vi "PhaseCalibration.vi"(0 "Global Parameters":T1={"DC AI Min (V)"=0.0015, "DC AI Max (V)"=0.06, "Mixer AI Min (V)"=-0.3, "Mixer AI Max (V)"=0.3, "Bias AO Min (V)"=-1.0, "Bias AO Max (V)"=7.0, "Scan AO Min (V)"=-10.0, "Scan AO Max (V)"=10.0, "Fast Samp Freq (Hz)"=2500000.0, "Slow Samp Freq (Hz)"=250000.0}, 1 "Bias Voltages":dbl[](array[numeric]), 2 "LaserRepRate":dbl=80000000.0, 5 "Calibration Parameters":T2={"Target Lifetime (s)"=4e-09, "Integration Time (s)"=0.1, "Calibration Steps"=500.0}, 7 "Mixer1 Values":dbl[](array[numeric]), 9 "Mixer2 Values":dbl[](array[numeric]), 11 "Mixer3 Values":dbl[](array[numeric]), 12 "Mixer4 Values":dbl[](array[numeric]), 13 "[V_DC]":dbl, 14 "[O_B]":dbl) -> (4 "Mixer Phases":cluster{"Bias voltage":dbl[], dbl[]}[](array[cluster]), 6 "Calibrated Bias Voltages":dbl[](array[numeric]) caption="Calibrated bias voltage", 8 "[M/B]":dbl, 10 "[V_IF_max]":dbl, 15 "[V_IF_min]":dbl)   [LabVIEW 2018]
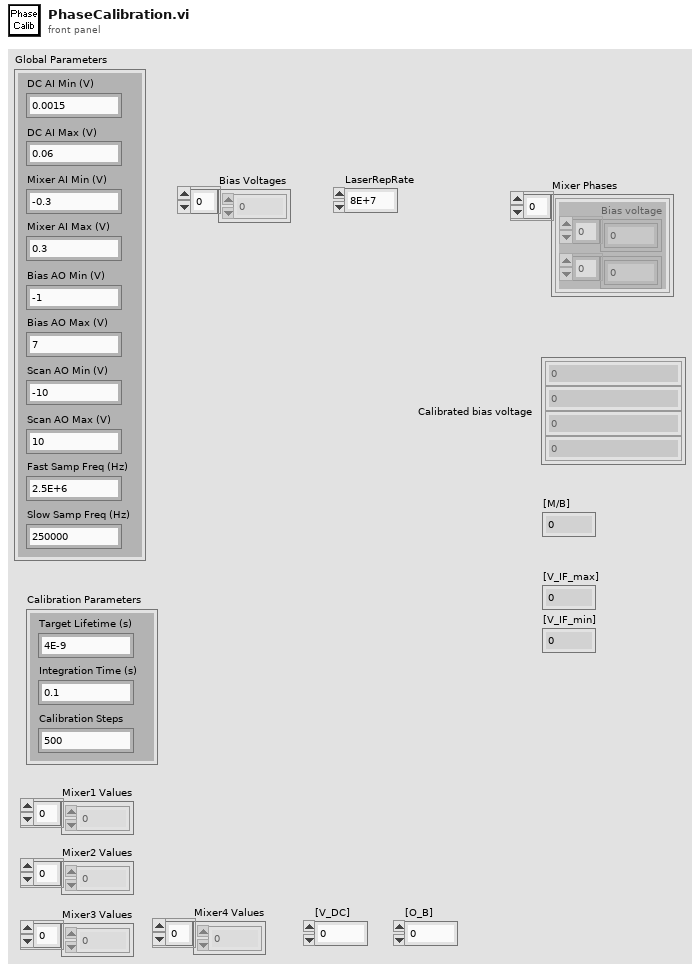
[diagram p1: front panel]
types:
  T1 = cluster{"DC AI Min (V)":dbl, "DC AI Max (V)":dbl, "Mixer AI Min (V)":dbl, "Mixer AI Max (V)":dbl, "Bias AO Min (V)":dbl, "Bias AO Max (V)":dbl, "Scan AO Min (V)":dbl, "Scan AO Max (V)":dbl, "Fast Samp Freq (Hz)":dbl, "Slow Samp Freq (Hz)":dbl}
  T2 = cluster{"Target Lifetime (s)":dbl, "Integration Time (s)":dbl, "Calibration Steps":dbl}
  T3 = cluster{"Bias Voltages":dbl[], "Phase Calibration Curve":dbl[]}
  T4 = cluster{"Bias Voltages":dbl[], "Phase Calibration Curve":dbl[]}[]
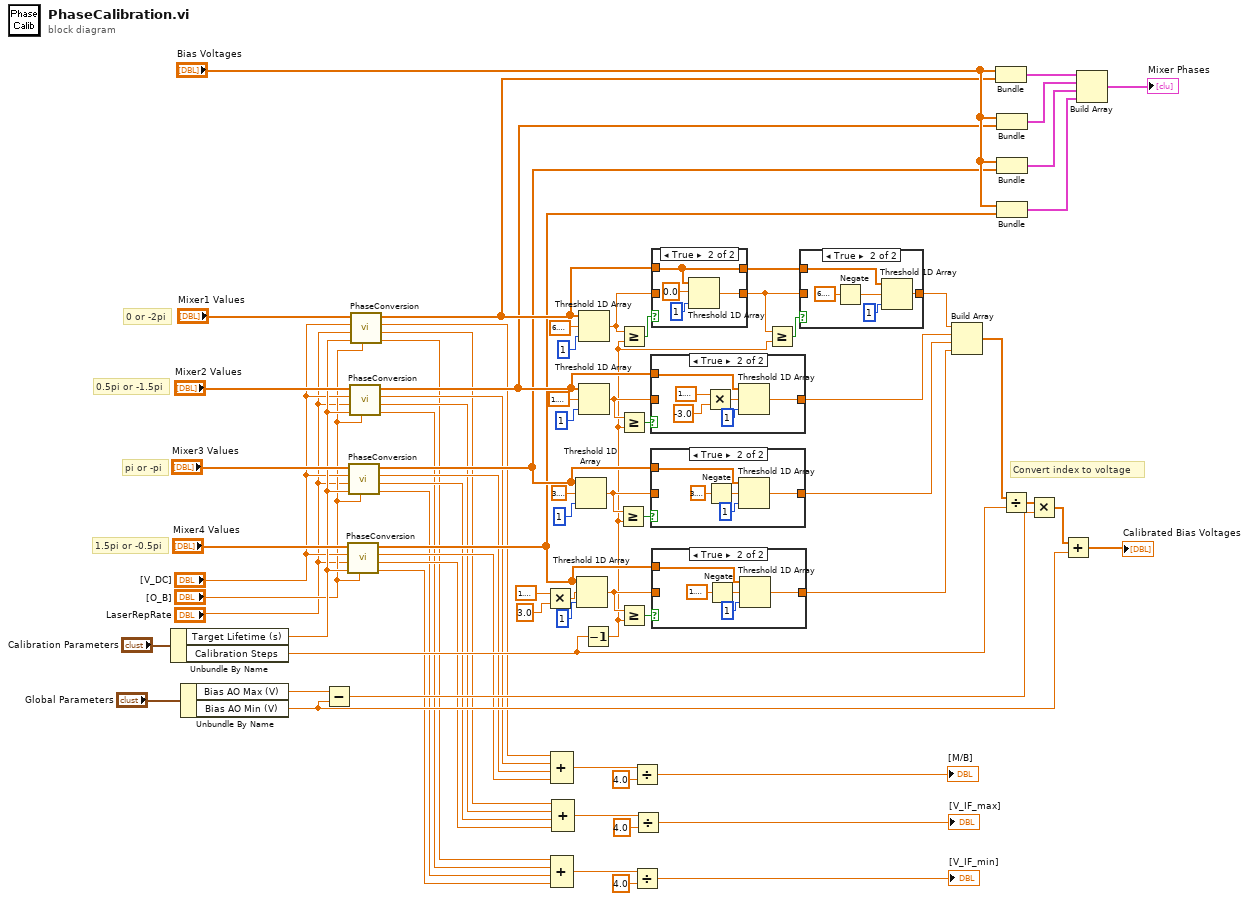
[diagram p0: block diagram]
diagram:
  # "Convert index to voltage"
  # "1.5pi or -0.5pi"
  # "pi or -pi"
  # "0.5pi or -1.5pi"
  # "0 or -2pi"
  n1 = Unbundle By Name("Calibration Parameters") -> ("Target Lifetime (s)"=w40:dbl, "Calibration Steps"=w61:dbl)
  n2 = Unbundle By Name("Global Parameters") -> ("Bias AO Max (V)"=w67:dbl, "Bias AO Min (V)"=w68:dbl)
  n3 = Subtract(x=w67, y=w68) -> (x-y=w72:dbl)
  n4 = call "PhaseConversion.vi"("[O_B]"="[O_B]", "Target Lifetime (s)"=w40, "Mod freq (Hz)"="LaserRepRate", "[V_DC]"="[V_DC]", "Mixer Values"="Mixer4 Values") -> ("V_IF_min"=w6:dbl, "V_IF_max"=w10:dbl, "M/B"=w27:dbl, "Phase Calibration Curve"=w41:dbl[])  [unwired: 2 in]
  n5 = call "PhaseConversion.vi"("[O_B]"="[O_B]", "Target Lifetime (s)"=w40, "Mod freq (Hz)"="LaserRepRate", "[V_DC]"="[V_DC]", "Mixer Values"="Mixer3 Values") -> ("V_IF_min"=w7:dbl, "V_IF_max"=w11:dbl, "M/B"=w26:dbl, "Phase Calibration Curve"=w42:dbl[])  [unwired: 2 in]
  n6 = call "PhaseConversion.vi"("[O_B]"="[O_B]", "Target Lifetime (s)"=w40, "Mod freq (Hz)"="LaserRepRate", "[V_DC]"="[V_DC]", "Mixer Values"="Mixer2 Values") -> ("V_IF_min"=w8:dbl, "V_IF_max"=w12:dbl, "M/B"=w25:dbl, "Phase Calibration Curve"=w43:dbl[])  [unwired: 2 in]
  n7 = call "PhaseConversion.vi"("[O_B]"="[O_B]", "Target Lifetime (s)"=w40, "Mod freq (Hz)"="LaserRepRate", "[V_DC]"="[V_DC]", "Mixer Values"="Mixer1 Values") -> ("V_IF_min"=w9:dbl, "V_IF_max"=w13:dbl, "M/B"=w24:dbl, "Phase Calibration Curve"=w44:dbl[])  [unwired: 2 in]
  n8 = Multiply(x=1.5707963267948966, y=3.0) -> (x*y=w57:dbl)
  n9 = Compound Arithmetic op=ADD(w24, w25, w26, w27) -> (w23:dbl)
  n10 = Compound Arithmetic op=ADD(w9, w8, w7, w6) -> (w15:dbl)
  n11 = Compound Arithmetic op=ADD(w13, w12, w11, w10) -> (w16:dbl)
  n12 = Threshold 1D Array(1:1 ("start index (0)"), 2:3.141592653589793, 3:w42) -> (0:w59:dbl)
  n13 = Threshold 1D Array(1:1 ("start index (0)"), 2:w57, 3:w41) -> (0:w53:dbl)
  n14 = Threshold 1D Array(1:1 ("start index (0)"), 2:6.283185307179586, 3:w44) -> (0:w49:dbl)
  n15 = Threshold 1D Array(1:1 ("start index (0)"), 2:1.5707963267948966, 3:w43) -> (0:w46:dbl)
  n16 = Decrement(x=w61) -> (x-1=w35:dbl)
  n17 = Greater Or Equal?(x=w59, y=w35) -> (x >= y?=w60:bool)
  n18 = Greater Or Equal?(x=w49, y=w35) -> (x >= y?=w50:bool)
  n19 = Greater Or Equal?(x=w46, y=w35) -> (x >= y?=w51:bool)
  n20 = Greater Or Equal?(x=w53, y=w35) -> (x >= y?=w54:bool)
  n21 = Divide(x=w23, y=4.0) -> (x/y=→"[M/B]":dbl)
  n22 = Divide(x=w15, y=4.0) -> (x/y=→"[V_IF_min]":dbl)
  n23 = Divide(x=w16, y=4.0) -> (x/y=→"[V_IF_max]":dbl)
  n24 = case shown="True" w51 {
    tunnel: [w76 w82] -> w45
    tunnel: w43 -> [_ w81]
    tunnel: w46 -> [w76 _]
    frame False {
    }
    frame True {
      n25 = Multiply(x=1.5707963267948966, y=-3.0) -> (x*y=w78:dbl)
      n26 = Threshold 1D Array(1:1 ("start index (0)"), 2:w78, 3:w81) -> (0:w82:dbl)
    }
  }
  n27 = case shown="True" w60 {
    tunnel: [w83 w88] -> w58
    tunnel: w59 -> [w83 _]
    tunnel: w42 -> [_ w85]
    frame False {
    }
    frame True {
      n28 = Negate(x=3.141592653589793) -> (-x=w87:dbl)
      n29 = Threshold 1D Array(1:1 ("start index (0)"), 2:w87, 3:w85) -> (0:w88:dbl)
    }
  }
  n30 = case shown="True" w50 {
    tunnel: [w90 w94] -> w34
    tunnel: w49 -> [w90 _]
    tunnel: w44 -> [w89 w92]
    tunnel: [w89 w92] -> w31
    frame False {
    }
    frame True {
      n31 = Threshold 1D Array(1:1 ("start index (0)"), 2:0.0 ("threshold y"), 3:w92) -> (0:w94:dbl)
    }
  }
  n32 = case shown="True" w54 {
    tunnel: [w95 w100] -> w52
    tunnel: w53 -> [w95 _]
    tunnel: w41 -> [_ w97]
    frame False {
    }
    frame True {
      n33 = Negate(x=1.5707963267948966) -> (-x=w99:dbl)
      n34 = Threshold 1D Array(1:1 ("start index (0)"), 2:w99, 3:w97) -> (0:w100:dbl)
    }
  }
  n35 = Greater Or Equal?(x=w34, y=w35) -> (x >= y?=w33:bool)
  n36 = case shown="True" w33 {
    tunnel: [w101 w106] -> w32
    tunnel: w34 -> [w101 _]
    tunnel: w31 -> [_ w104]
    frame False {
    }
    frame True {
      n37 = Negate(x=6.283185307179586) -> (-x=w102:dbl)
      n38 = Threshold 1D Array(1:1 ("start index (0)"), 2:w102, 3:w104) -> (0:w106:dbl)
    }
  }
  n39 = Build Array(w32, w45, w58, w52) -> (w29:dbl[])
  n40 = Bundle("Bias Voltages"="Bias Voltages", "Phase Calibration Curve"=w44) -> (w75:T3)  [unwired: 1 in]
  n41 = Bundle("Bias Voltages"="Bias Voltages", "Phase Calibration Curve"=w43) -> (w20:T3)  [unwired: 1 in]
  n42 = Bundle("Bias Voltages"="Bias Voltages", "Phase Calibration Curve"=w42) -> (w19:T3)  [unwired: 1 in]
  n43 = Bundle("Bias Voltages"="Bias Voltages", "Phase Calibration Curve"=w41) -> (w18:T3)  [unwired: 1 in]
  n44 = Divide(x=w29, y=w61) -> (x/y=w74:dbl[])
  n45 = Multiply(x=w74, y=w72) -> (x*y=w73:dbl[])
  n46 = Add(x=w73, y=w68) -> (x+y=→"Calibrated Bias Voltages":dbl[])
  n47 = Build Array(w75, w20, w19, w18) -> (→"Mixer Phases":T4)
